vi "Peak Detection (Wavelet vs. Normal).vi"() -> ()   [LabVIEW 2023]
doc: "This example compares the wavelet transform-based peak detection method with the traditional curve fitting-based method. The wavelet transform-based method is more robust and accurate. This example uses the WA Multiscale Peak Detection VI and the Peak Detector VI for the wavelet transform-based and the curve fitting-based methods, respectively.\n\n<b>Instructions:</b>\n1) Run this VI.\n2) Compare the peak detection results of the wavelet transform-based and the curve fitting-based methods.\n3) Drag the cursors to set thresholds for the peaks and valleys."
uses:
  <vilib>/Analysis/1siggen.llb/Ramp Pattern by Samples.vi
  <vilib>/addons/Wavelet Analysis/application.llb/WA Multiscale Peak Detection (Array).vi
  <vilib>/Analysis/NI_AALBase.lvlib
  <vilib>/addons/_Advanced Signal Processing/NI_AdvSigProcWA.lvlib
  <vilib>/Analysis/NI_AAL_SigProc.lvlib
panel:
  in  "stop":bool
  in  "Width":i32=8
  out "display":T1(graph)
  # "Overview: Compares the wavelet transform-based peak detection method with the traditional curve fitting-based method. \nRequirements: LabVIEW Full Development System, Advanced Signal Processing Toolkit\nInstructions: \n1. Run this VI.\n2. Compare the peak detection results of the wavelet transform-based and the curve fitting-based methods.\n3. Drag the cursors to set thresholds for the peaks and valleys.\n4. Click Stop to stop the VI."
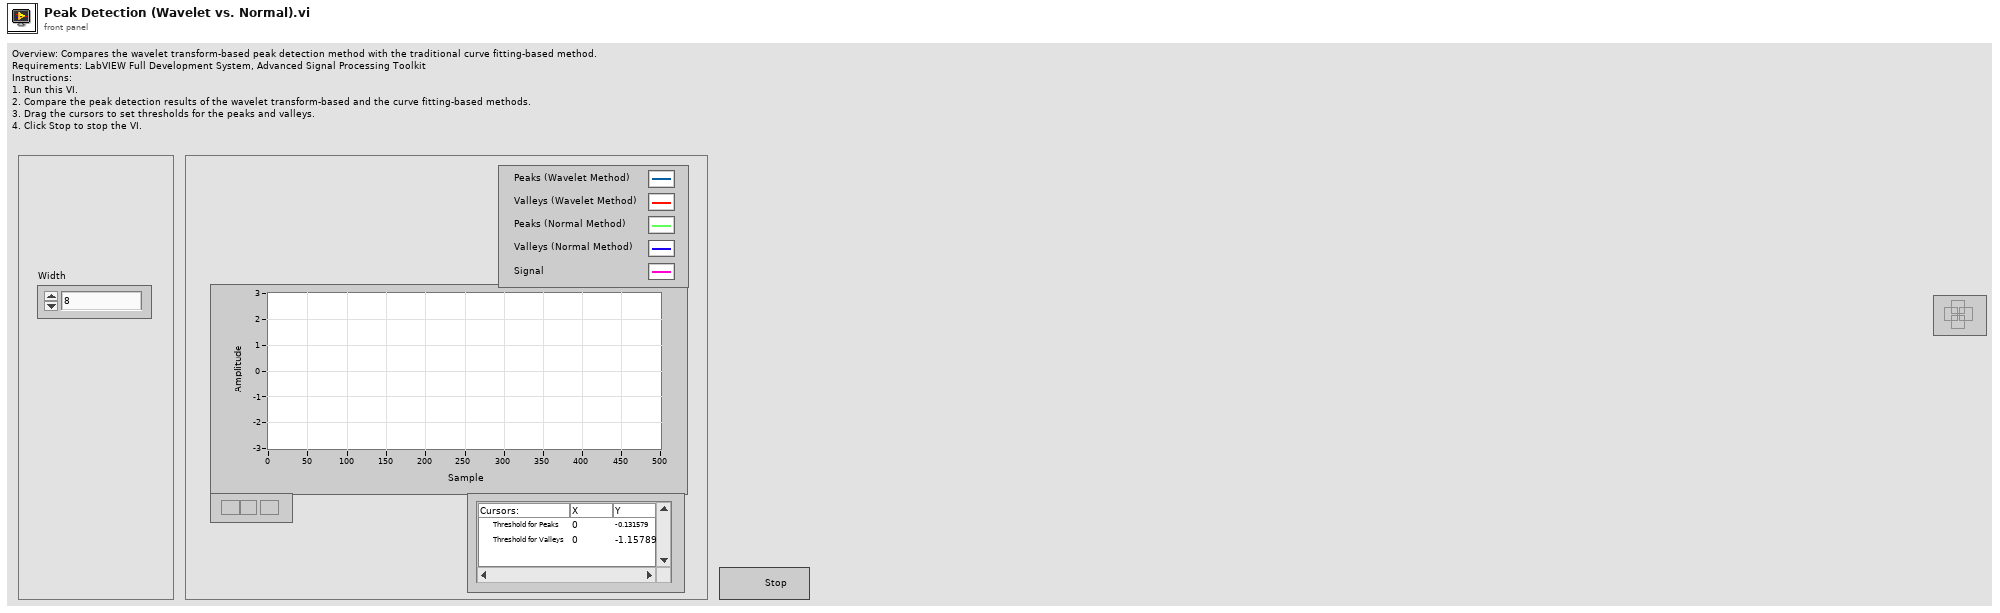
[diagram p1: front panel]
types:
  T1 = cluster{"Ramp Pattern":dbl[], "Amplitudes":dbl[]}[]
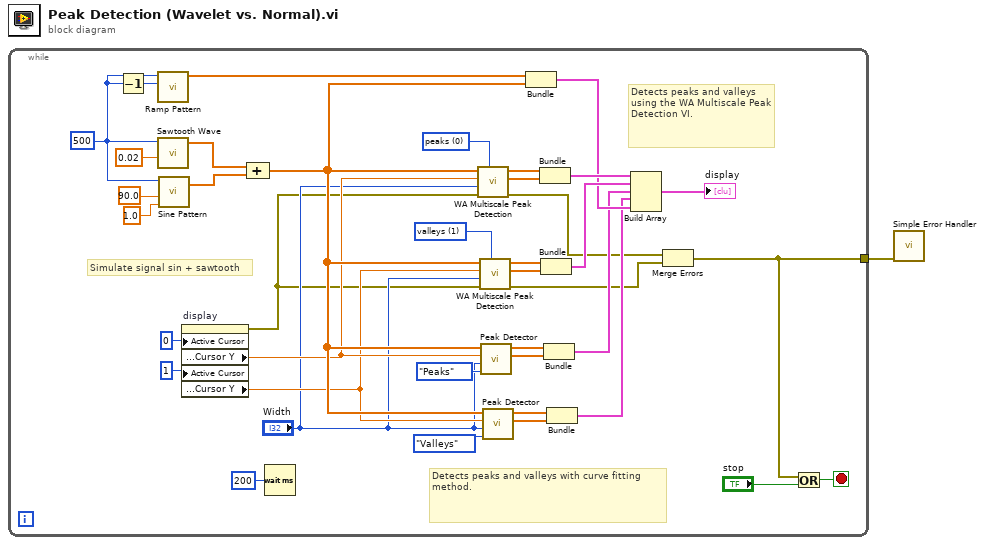
[diagram p0: block diagram]
diagram:
  n1 = while {
    tunnel: [w3] -> w1
    stop <- w5 stop-if-true
    w33 = u16 1 items=["peaks", "valleys"] ("peaks/valleys")
    w34 = u16 0 items=["peaks", "valleys"] ("peaks/valleys")
    w10 = 500 ("samples")
    # "Detects peaks and valleys with curve fitting method."
    # "Detects peaks and valleys using the WA Multiscale Peak Detection VI."
    # "Simulate signal sin + sawtooth"
    n2 = Decrement(x=w10) -> (x-1=w32:i32)
    n3 = call-poly <vilib>:"Ramp Pattern.vi"("end"=w32, "samples"=w10) -> ("Ramp Pattern"=w31:dbl[])  [unwired: 8 in, 1 out]
    n4 = call <vilib>:"Sawtooth Wave.vi"("samples"=w10, "frequency"=0.02 ("f")) -> ("sawtooth wave"=w38:dbl[])  [unwired: 3 in, 2 out]
    n5 = call <vilib>:"Sine Pattern.vi"("cycles"=1.0, "phase(degrees)"=90.0, "samples"=w10) -> ("Sinusoidal Pattern"=w37:dbl[])  [unwired: 1 in, 1 out]
    n6 = property on="display" class="XYGraph (strict)"("Active Cursor"=u32 0, "Active Cursor"=u32 1) -> (error out=w2:errorcluster, "Cursor.Cursor Position:Cursor Y"=w22:dbl, "Cursor.Cursor Position:Cursor Y"=w21:dbl)  [unwired: 2 in, 1 out]
    n7 = Compound Arithmetic op=ADD(w38, w37) -> (w23:dbl[])
    n8 = Wait (ms)(milliseconds to wait=u32 200 ("millisecond multiple")) -> ()  [unwired: 1 out]
    n9 = call-poly <vilib>:"WA Multiscale Peak Detection.vi"("peaks/valleys"=w34, "error in (no error)"=w2, "width"="Width", "threshold"=w22, "signal"=w23) -> ("error out"=w8:errorcluster, "amplitude"=w29:dbl[], "location"=w30:dbl[])  [unwired: 2 in, 2 out]
    n10 = call-poly <vilib>:"WA Multiscale Peak Detection.vi"("peaks/valleys"=w33, "error in (no error)"=w2, "width"="Width", "threshold"=w21, "signal"=w23) -> ("error out"=w7:errorcluster, "amplitude"=w27:dbl[], "location"=w28:dbl[])  [unwired: 2 in, 2 out]
    n11 = call <vilib>:"Peak Detector.vi"("peaks/valleys"=enum32{"Peaks", "Valleys"}."Peaks", "width"="Width", "threshold"=w22, "X"=w23) -> ("Amplitudes"=w16:dbl[], "Locations"=w17:dbl[])  [unwired: 3 in, 3 out]
    n12 = call <vilib>:"Peak Detector.vi"("peaks/valleys"=enum32{"Peaks", "Valleys"}."Valleys", "width"="Width", "threshold"=w21, "X"=w23) -> ("Amplitudes"=w14:dbl[], "Locations"=w15:dbl[])  [unwired: 3 in, 3 out]
    n13 = Bundle("Ramp Pattern"=w31, w23) -> (w13:cluster{"Ramp Pattern":dbl[], dbl[]})  [unwired: 1 out]
    n14 = Bundle("location"=w30, "amplitude"=w29) -> (w26:cluster{"location":dbl[], "amplitude":dbl[]})  [unwired: 1 out]
    n15 = Bundle("location"=w28, "amplitude"=w27) -> (w25:cluster{"location":dbl[], "amplitude":dbl[]})  [unwired: 1 out]
    n16 = Bundle("Locations"=w17, "Amplitudes"=w16) -> (w12:cluster{"Locations":dbl[], "Amplitudes":dbl[]})  [unwired: 1 out]
    n17 = Bundle("Locations"=w15, "Amplitudes"=w14) -> (w11:cluster{"Locations":dbl[], "Amplitudes":dbl[]})  [unwired: 1 out]
    n18 = Build Array(w26, w25, w12, w11, w13) -> (→"display":T1)
    n19 = Merge Errors(w8, w7) -> (w3:errorcluster)
    n20 = Or(x=w3, y="stop") -> (x .or. y?=w5:bool)
  }
  n21 = call <vilib>:"Simple Error Handler.vi"("error in (no error)"=w1) -> ()  [unwired: 1 in, 8 out]
